vi "tolerance calculator.vi"(10 "Set point":dbl, 11 "Tolerance":dbl) -> (3 "output cluster":cluster{"upper limit":dbl, "lower limit":dbl})   [LabVIEW 2019]
panel:
  in  "ALIMENTATORE VARIAC":T1={"STATO"={"Comunicazione"=FALSE, "Abilitato"=FALSE, "RUNNING"=FALSE, "ALLARME"=FALSE, "FINE RAMPA"=FALSE}, "START\\STOP"={"START"=FALSE, "STOP"=FALSE}, "SETPOINT"={"TENSIONE [V]"=0.0, "Rampa tensione"=0.0, "PID V"=FALSE, "PID F"=FALSE, "SET V F"=FALSE}, "connetti"={"Comunicazione"=FALSE, "Connetti"=FALSE, "Disconnetti"=FALSE}, "Stato config"={"RPM"=0.0, "Vnom"=0.0, "HZnom"=0.0, "Inom"=0.0, "kWnom"=0.0, "TipoMot."=0.0}, "Controlli"={"Trampa[s]"=10.0, "Stato rampa"=10.0, "Inverti senso di rotazione"=FALSE}, "Config"=FALSE} {"Controlli"."Trampa[s]" min=0.1; "SETPOINT"."Rampa tensione" scale=0.0..500.0}
  # "~ ALIMENTATORE VARIAC~"
  # "CONNESSIONE..."
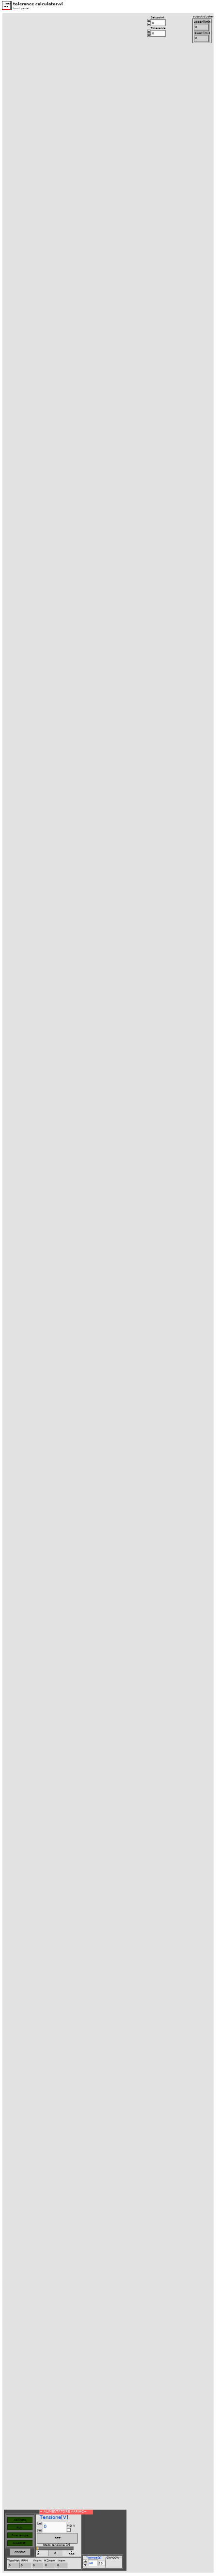
[diagram p1: front panel]
types:
  T1 = cluster{"STATO":cluster{"Comunicazione":bool, "Abilitato":bool, "RUNNING":bool, "ALLARME":bool, "FINE RAMPA":bool}, "START\\STOP":cluster{"START":bool, "STOP":bool}, "SETPOINT":cluster{"TENSIONE [V]":dbl, "Rampa tensione":dbl, "PID V":bool, "PID F":bool, "SET V F":bool}, "connetti":cluster{"Comunicazione":bool, "Connetti":bool, "Disconnetti":bool}, "Stato config":cluster{"RPM":dbl, "Vnom":dbl, "HZnom":dbl, "Inom":dbl, "kWnom":dbl, "TipoMot.":dbl}, "Controlli":cluster{"Trampa[s]":dbl, "Stato rampa":dbl, "Inverti senso di rotazione":bool}, "Config":bool}
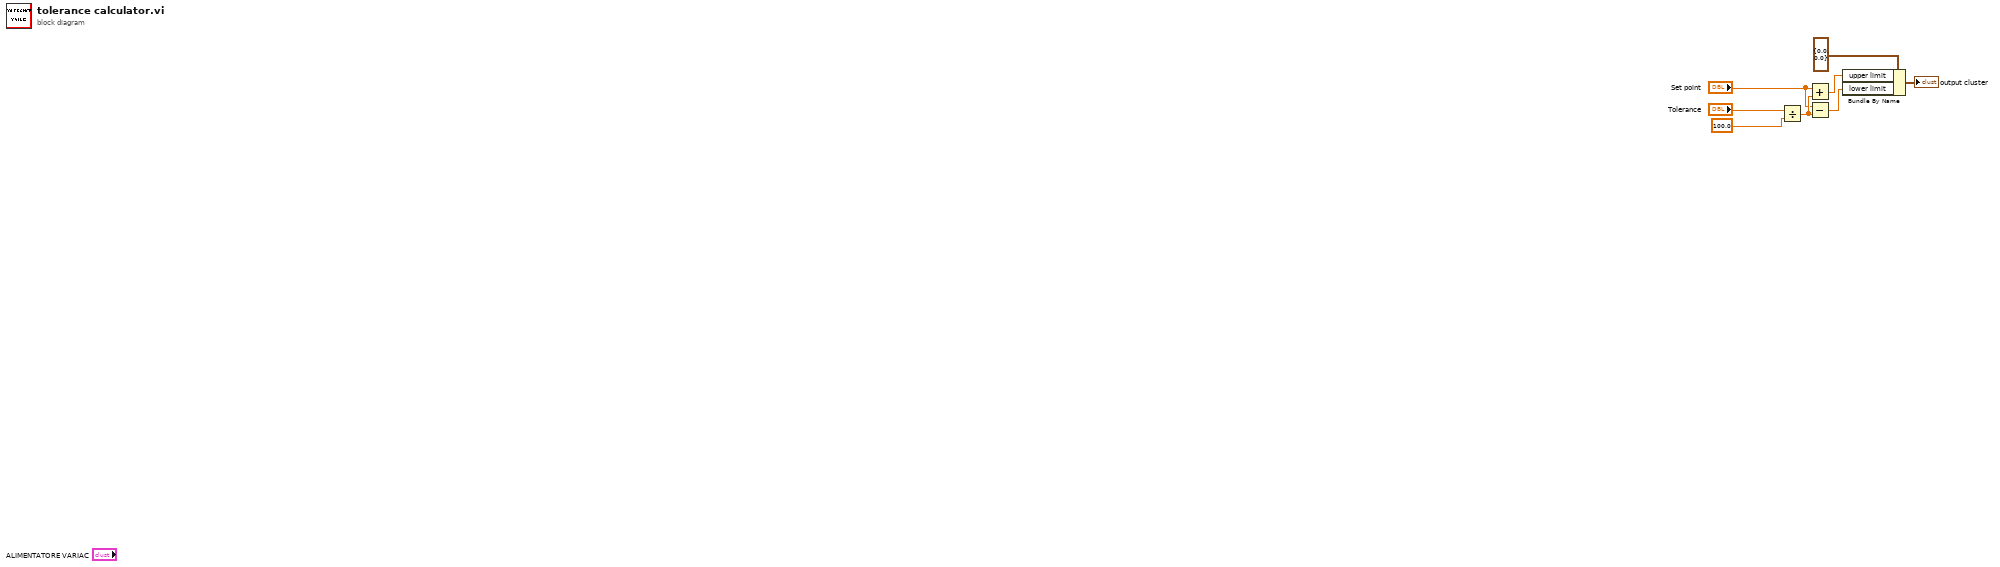
[diagram p0: block diagram]
diagram:
  n1 = Divide(x="Tolerance", y=100.0) -> (x/y=w6:dbl)
  n2 = Add(x="Set point", y=w6) -> (x+y=w7:dbl)
  n3 = Subtract(x="Set point", y=w6) -> (x-y=w8:dbl)
  n4 = Bundle By Name(cluster=cluster{"upper limit":dbl, "lower limit":dbl} {"upper limit"=0.0, "lower limit"=0.0}, "upper limit"=w7, "lower limit"=w8) -> (→"output cluster":cluster{"upper limit":dbl, "lower limit":dbl})
